vi "Read UDP Message.vi"(8 "error in":errorcluster, 11 "Local UDP connection ref":refnum<k16>) -> (0 "error out":errorcluster, 2 "data out":string, 3 "Local UDP connection ref out":refnum<k16>, 4 "Remote IP":string, 6 "Remote Port":u16)   [LabVIEW 2021, in "UDP Comms.lvlib"]
uses:
  UDP Comms.lvlib
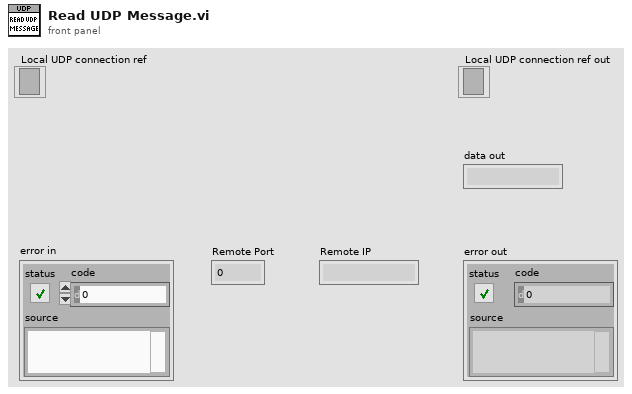
[diagram p1: front panel]
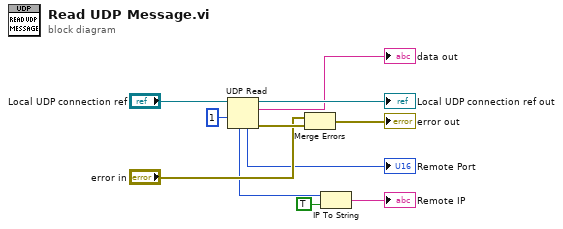
[diagram p0: block diagram]
diagram:
  n1 = UDP Read(connection ID="Local UDP connection ref", timeout ms (25000)=1) -> (data out=→"data out":string, error out=w10:errorcluster, 3:→"Local UDP connection ref out":refnum<k16>, 4:→"Remote Port":u16, 6:w6:u32)  [unwired: 2 in]
  n2 = Merge Errors("error in", w10) -> (→"error out":errorcluster)
  n3 = IP To String(1:TRUE ("dot notation? (F)"), 2:w6) -> (0:→"Remote IP":string)
